vi "ep_Check Speed Nameplate.vi"(7 "check? (F)":bool, 8 "error in (no error)":errorcluster, 11 "nameplate information":T1) -> (0 "error out":errorcluster)   [LabVIEW 2014, in "NI_EP_Motor Monitoring.lvlib"]
uses:
  <vilib>/addons/Electrical Power/Motor Monitoring/NI_EP_Motor Monitoring.lvlib
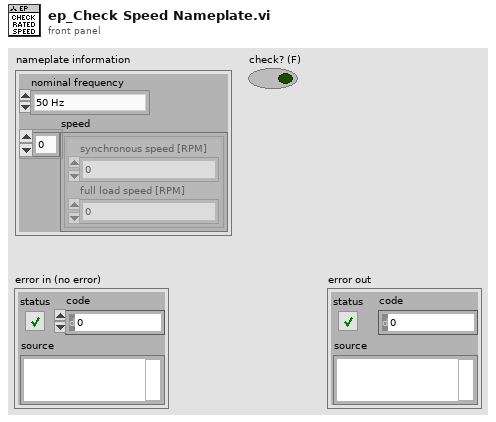
[diagram p1: front panel]
types:
  T1 = cluster{"nominal frequency":enum16{"50 Hz", "60 Hz"}, "speed":cluster{"synchronous speed [RPM]":dbl, "full load speed [RPM]":dbl}[]}
  T2 = cluster{"synchronous speed [RPM]":dbl, "full load speed [RPM]":dbl}[]
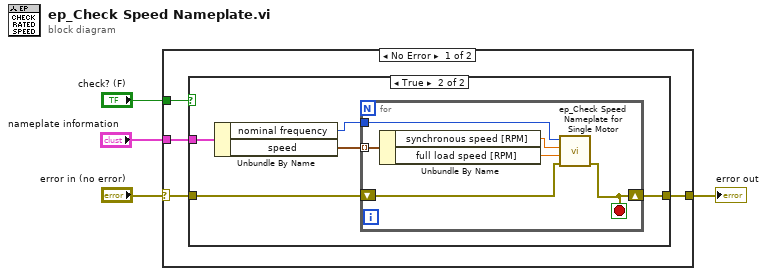
[diagram p0: block diagram]
diagram:
  n1 = case shown="No Error" "error in (no error)" {
    selector: "error in (no error)" -> [w6 w21]
    tunnel: [w7 w21] -> w3
    tunnel: "nameplate information" -> [w8 _]
    tunnel: "check? (F)" -> [w5 _]
    frame No Error {
      n2 = case shown="True" w5 {
        tunnel: w8 -> [_ w12]
        tunnel: [w9 w14] -> w7
        tunnel: w6 -> [w9 w13]
        frame False {
        }
        frame True {
          n3 = Unbundle By Name(w12) -> ("nominal frequency"=w10:enum16{"50 Hz", "60 Hz"}, "speed"=w11:T2)
          n4 = for {
            tunnel: w11 -> [w20] mode=indexing
            shift-right: [w15] -> w14
            shift-left: w13 -> [w16]
            tunnel: w10 -> [w19]
            stop <- w15 stop-if-true
            n5 = Unbundle By Name(w20) -> ("synchronous speed [RPM]"=w17:dbl, "full load speed [RPM]"=w18:dbl)
            n6 = call <vilib>:"ep_Check Speed Nameplate for Single Motor.vi"("error in (no error)"=w16, "full load speed [RPM]"=w18, "synchronous speed [RPM]"=w17, "nominal frequency"=w19) -> ("error out"=w15:errorcluster)  [unwired: 7 in]
          }
        }
      }
    }
    frame Error {
    }
  }
  "error out" <- w3
